vi "Get specification tolerances.vi"(8 "error in (no error)":errorcluster, 11 "VISA resource name":refnum<visa-resource-name>) -> (0 "error out":errorcluster, 1 "24 hour string":string, 2 "24 hours":dbl, 3 "VISA resource name out":refnum<visa-resource-name>, 4 "1 year string":string, 5 "90 days string":string, 6 "1 year":dbl, 7 "90 days":dbl)   [LabVIEW 2012, in "Datron D4xxx.lvlib"]
doc: "This VI returns specification tolerances (P0 to P2 commands)."
uses:
  Datron D4xxx.lvlib
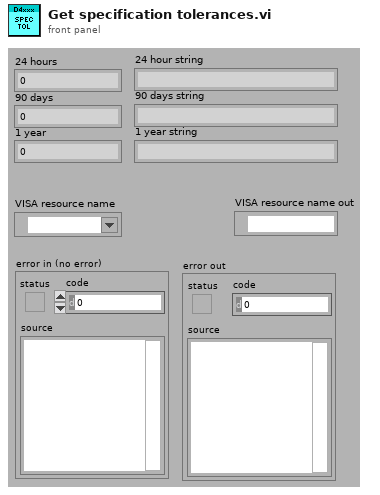
[diagram p1: front panel]
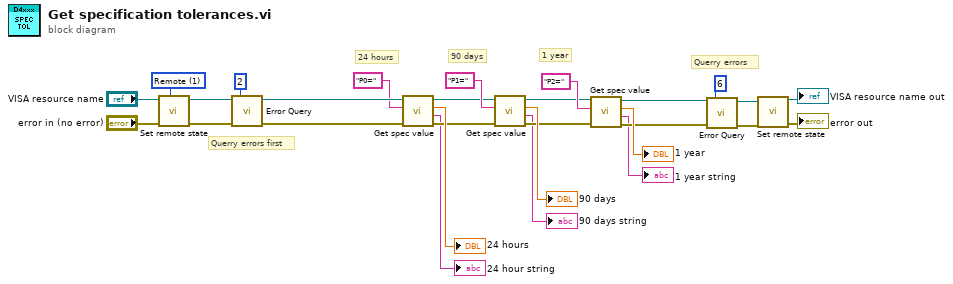
[diagram p0: block diagram]
diagram:
  w26 = u16 1 items=["Local", "Remote", "Default"] ("Remote state")
  # "Querry errors"
  # "1 year"
  # "90 days"
  # "Querry errors first"
  # "24 hours"
  n1 = call "Set remote state.vi"("error in"="error in (no error)", "Remote state"=w26, "VISA resource name"="VISA resource name") -> ("error out"=w23:errorcluster, "VISA resource name out"=w22:refnum<visa-resource-name>)  [unwired: 7 in]
  n2 = call "Error Query.vi"("error in (no error)"=w23, "Check cycles (11)"=2, "VISA resource name"=w22) -> ("error out"=w20:errorcluster, "VISA resource name out"=w19:refnum<visa-resource-name>)  [unwired: 5 in, 2 out]
  n3 = call "Get spec value.vi"("error in (no error)"=w20, "Command string"="P0=" ("write buffer"), "VISA resource name"=w19) -> ("error out"=w12:errorcluster, "Value string"=→"24 hour string":string, "Value"=→"24 hours":dbl, "VISA resource name out"=w10:refnum<visa-resource-name>)  [unwired: 5 in]
  n4 = call "Get spec value.vi"("error in (no error)"=w12, "Command string"="P1=" ("write buffer"), "VISA resource name"=w10) -> ("error out"=w11:errorcluster, "Value string"=→"90 days string":string, "Value"=→"90 days":dbl, "VISA resource name out"=w9:refnum<visa-resource-name>)  [unwired: 5 in]
  n5 = call "Get spec value.vi"("error in (no error)"=w11, "Command string"="P2=" ("write buffer"), "VISA resource name"=w9) -> ("error out"=w8:errorcluster, "Value string"=→"1 year string":string, "Value"=→"1 year":dbl, "VISA resource name out"=w7:refnum<visa-resource-name>)  [unwired: 5 in]
  n6 = call "Error Query.vi"("error in (no error)"=w8, "Check cycles (11)"=6, "VISA resource name"=w7) -> ("error out"=w4:errorcluster, "VISA resource name out"=w5:refnum<visa-resource-name>)  [unwired: 5 in, 2 out]
  n7 = call "Set remote state.vi"("error in"=w4, "VISA resource name"=w5) -> ("error out"=→"error out":errorcluster, "VISA resource name out"=→"VISA resource name out":refnum<visa-resource-name>)  [unwired: 8 in]
